vi "hmi_shutdown.vi"(7 "references":T1, 8 "error in (no error)":errorcluster) -> (0 "error out":errorcluster)   [LabVIEW 2015, in "lv-dialog-interfaces.lvlib"]
uses:
  lv-dialog-interfaces.lvlib
  _controls/hmi_references.ctl
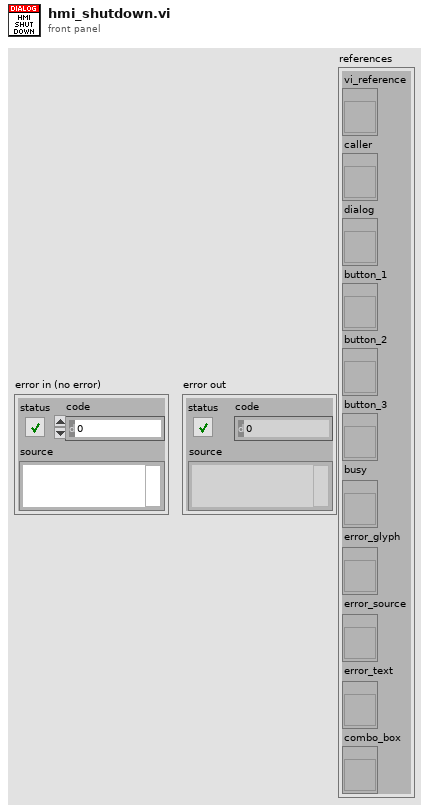
[diagram p1: front panel]
types:
  T1 = typedef "lv-dialog-interfaces.lvlib/hmi_references.ctl" = cluster{"vi_reference":refnum<vi>, "caller":refnum<vi>, "dialog":refnum<vi>, "button_1":refnum<vi>, "button_2":refnum<vi>, "button_3":refnum<vi>, "busy":refnum<vi>, "error_glyph":refnum<vi>, "error_source":refnum<vi>, "error_text":refnum<vi>, "combo_box":refnum<vi>}
  T2 = typedef "LVRectTypeDef.ctl" = cluster{"Left":i16, "Top":i16, "Right":i16, "Bottom":i16}
  T3 = typedef "LVPointTypeDef.ctl" = cluster{"Horizontal":i16, "Vertical":i16}
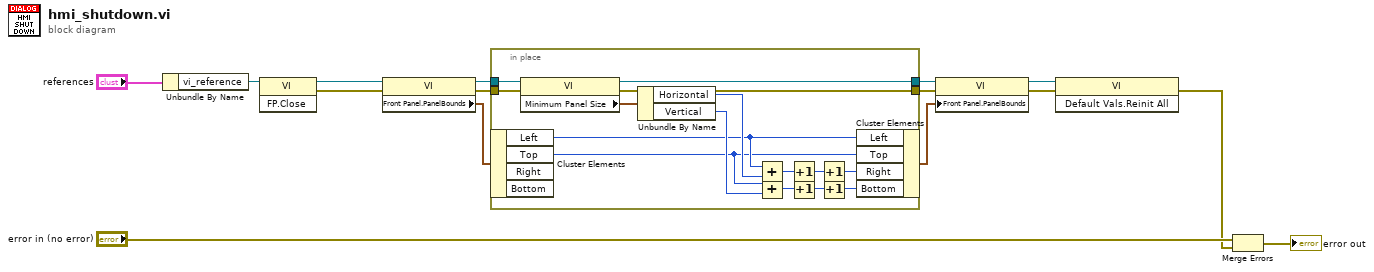
[diagram p0: block diagram]
diagram:
  n1 = Unbundle By Name("references") -> ("vi_reference"=w12:refnum<vi>)
  n2 = invoke class="VI" method="FP.Close"(reference=w12) -> (reference out=w10:refnum<vi>, error out=w9:errorcluster)  [unwired: 2 in, 1 out]
  n3 = property class="VI"(reference=w10, error in=w9) -> (reference out=w4:refnum<vi>, error out=w3:errorcluster, "Front Panel.PanelBounds"=w6:T2)
  n4 = in-place {
    in-place-border: w4 -> [w30]
    in-place-border: w3 -> [w29]
    in-place-border: [w28] -> w2
    in-place-border: [w27] -> w1
    n5 = in-place-cluster #1(w6) -> ("Left"=w20:i16, "Top"=w18:i16)  [unwired: 2 out]
    n6 = property class="VI"(reference=w30, error in=w29) -> (reference out=w28:refnum<vi>, error out=w27:errorcluster, "Minimum Panel Size"=w26:T3)
    n7 = Unbundle By Name(w26) -> ("Horizontal"=w23:i16, "Vertical"=w22:i16)
    n8 = Add(x=w20, y=w23) -> (x+y=w25:i16)
    n9 = Add(x=w18, y=w22) -> (x+y=w24:i16)
    n10 = Increment(x=w25) -> (x+1=w21:i16)
    n11 = Increment(x=w24) -> (x+1=w19:i16)
    n12 = Increment(x=w21) -> (x+1=w17:i16)
    n13 = Increment(x=w19) -> (x+1=w16:i16)
    n14 = in-place-cluster #1("Left"=w20, "Top"=w18, "Right"=w17, "Bottom"=w16) -> (w5:T2)
  }
  n15 = property class="VI"(reference=w2, error in=w1, "Front Panel.PanelBounds"=w5) -> (reference out=w7:refnum<vi>, error out=w8:errorcluster)
  n16 = invoke class="VI" method="Default Vals.Reinit All"(reference=w7, error in=w8) -> (error out=w11:errorcluster)  [unwired: 1 in, 2 out]
  n17 = Merge Errors("error in (no error)", w11) -> (→"error out":errorcluster)
